vi "Przenies param rej wolna FVG.vi"(7 "Wolna In":T1={"WolnaStart"=FALSE, "WolnaPrzeglad"=FALSE, "Okres"=0.02, "Czas max"=120.0, "WolnaKonfiguracja"=FALSE, "Rej.1"={"Typ rejestracji"=enum."Wprost", "Kanały"=[1], "Opis"="Rej.X", "Aktywny"=FALSE, "Wolna Wykr num"=0}, "Rej.2"={"Typ rejestracji"=enum."Wprost", "Kanały"=[1], "Opis"="Rej.X", "Aktywny"=FALSE, "Wolna Wykr num"=0}, "Rej.3"={"Typ rejestracji"=enum."Wprost", "Kanały"=[1], "Opis"="Rej.X", "Aktywny"=FALSE, "Wolna Wykr num"=0}, "Rej.4"={"Typ rejestracji"=enum."Wprost", "Kanały"=[1], "Opis"="Rej.X", "Aktywny"=FALSE, "Wolna Wykr num"=0}, "Rej.5"={"Typ rejestracji"=enum."Wprost", "Kanały"=[1], "Opis"="Rej.X", "Aktywny"=FALSE, "Wolna Wykr num"=0}, "Rej.6"={"Typ rejestracji"=enum."Wprost", "Kanały"=[1], "Opis"="Rej.X", "Aktywny"=FALSE, "Wolna Wykr num"=0}, "Rej.7"={"Typ rejestracji"=enum."Wprost", "Kanały"=[1], "Opis"="Rej.X", "Aktywny"=FALSE, "Wolna Wykr num"=0}, "Rej.8"={"Typ rejestracji"=enum."Wprost", "Kanały"=[1], "Opis"="Rej.X", "Aktywny"=FALSE, "Wolna Wykr num"=0}} {"Rej.8"."Wolna Wykr num" items=["Brak", "Wykres 1", "Wykres 2", "Wykres 3", "Wykres 4"]; "Rej.7"."Wolna Wykr num" items=["Brak", "Wykres 1", "Wykres 2", "Wykres 3", "Wykres 4"]; "Rej.6"."Wolna Wykr num" items=["Brak", "Wykres 1", "Wykres 2", "Wykres 3", "Wykres 4"]; "Rej.5"."Wolna Wykr num" items=["Brak", "Wykres 1", "Wykres 2", "Wykres 3", "Wykres 4"]; "Rej.4"."Wolna Wykr num" items=["Brak", "Wykres 1", "Wykres 2", "Wykres 3", "Wykres 4"]; "Rej.3"."Wolna Wykr num" items=["Brak", "Wykres 1", "Wykres 2", "Wykres 3", "Wykres 4"]; "Rej.2"."Wolna Wykr num" items=["Brak", "Wykres 1", "Wykres 2", "Wykres 3", "Wykres 4"]; "Rej.1"."Wolna Wykr num" items=["Brak", "Wykres 1", "Wykres 2", "Wykres 3", "Wykres 4"]}, 8 "error in (no error)":errorcluster, 10 "Start In":bool, 11 "Akcja":T5) -> (0 "error out":errorcluster, 2 "Start Out":bool, 3 "Restart Out":bool, 6 "Wolna Out":T1={"WolnaStart"=FALSE, "WolnaPrzeglad"=FALSE, "Okres"=0.02, "Czas max"=120.0, "WolnaKonfiguracja"=FALSE, "Rej.1"={"Typ rejestracji"=enum."Wprost", "Kanały"=[1], "Opis"="Rej.X", "Aktywny"=FALSE, "Wolna Wykr num"=0}, "Rej.2"={"Typ rejestracji"=enum."Wprost", "Kanały"=[1], "Opis"="Rej.X", "Aktywny"=FALSE, "Wolna Wykr num"=0}, "Rej.3"={"Typ rejestracji"=enum."Wprost", "Kanały"=[1], "Opis"="Rej.X", "Aktywny"=FALSE, "Wolna Wykr num"=0}, "Rej.4"={"Typ rejestracji"=enum."Wprost", "Kanały"=[1], "Opis"="Rej.X", "Aktywny"=FALSE, "Wolna Wykr num"=0}, "Rej.5"={"Typ rejestracji"=enum."Wprost", "Kanały"=[1], "Opis"="Rej.X", "Aktywny"=FALSE, "Wolna Wykr num"=0}, "Rej.6"={"Typ rejestracji"=enum."Wprost", "Kanały"=[1], "Opis"="Rej.X", "Aktywny"=FALSE, "Wolna Wykr num"=0}, "Rej.7"={"Typ rejestracji"=enum."Wprost", "Kanały"=[1], "Opis"="Rej.X", "Aktywny"=FALSE, "Wolna Wykr num"=0}, "Rej.8"={"Typ rejestracji"=enum."Wprost", "Kanały"=[1], "Opis"="Rej.X", "Aktywny"=FALSE, "Wolna Wykr num"=0}} {"Rej.8"."Wolna Wykr num" items=["Brak", "Wykres 1", "Wykres 2", "Wykres 3", "Wykres 4"]; "Rej.7"."Wolna Wykr num" items=["Brak", "Wykres 1", "Wykres 2", "Wykres 3", "Wykres 4"]; "Rej.6"."Wolna Wykr num" items=["Brak", "Wykres 1", "Wykres 2", "Wykres 3", "Wykres 4"]; "Rej.5"."Wolna Wykr num" items=["Brak", "Wykres 1", "Wykres 2", "Wykres 3", "Wykres 4"]; "Rej.4"."Wolna Wykr num" items=["Brak", "Wykres 1", "Wykres 2", "Wykres 3", "Wykres 4"]; "Rej.3"."Wolna Wykr num" items=["Brak", "Wykres 1", "Wykres 2", "Wykres 3", "Wykres 4"]; "Rej.2"."Wolna Wykr num" items=["Brak", "Wykres 1", "Wykres 2", "Wykres 3", "Wykres 4"]; "Rej.1"."Wolna Wykr num" items=["Brak", "Wykres 1", "Wykres 2", "Wykres 3", "Wykres 4"]})   [LabVIEW 2013]
doc: "Use this template to build a VI to use as a subVI."
uses:
  Kontrolki/FVGs/FVG akwizycje akcje.ctl
  Kontrolki/GUI/Rejestracja_wolna.ctl
  Kontrolki/GUI/RejWol_konfig.ctl
  Kontrolki/GUI/RejWol_typ.ctl
  Kontrolki/GUI/Wolna_WykrNum.ctl
panel:
  out "Śledzenie Out":enum16{"Obwiednia", "Migawka"}(ring)
  in  "Śledzenie In":enum16{"Obwiednia", "Migawka"}(ring)
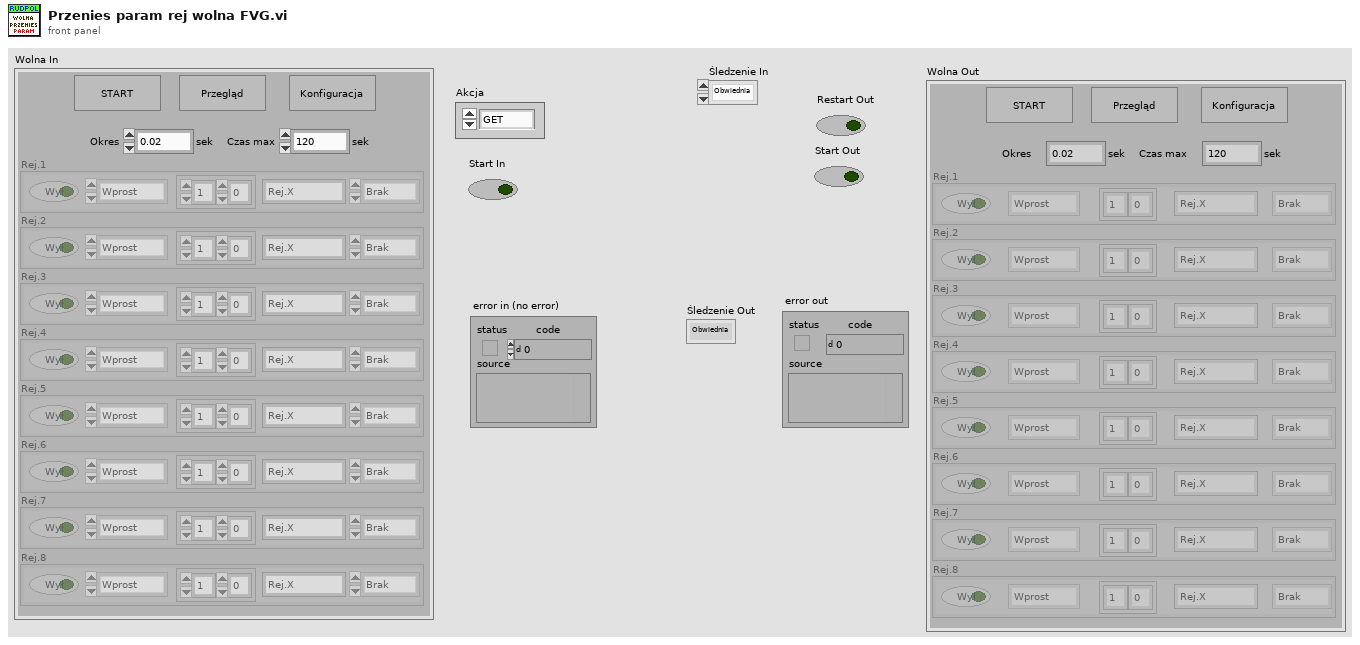
[diagram p1: front panel]
types:
  T1 = typedef "Rejestracja_wolna.ctl" = cluster{"WolnaStart":bool, "WolnaPrzeglad":bool, "Okres":dbl, "Czas max":dbl, "WolnaKonfiguracja":bool, "Rej.1":T2, "Rej.2":T2, "Rej.3":T2, "Rej.4":T2, "Rej.5":T2, "Rej.6":T2, "Rej.7":T2, "Rej.8":T2}
  T2 = typedef "RejWol_konfig.ctl" = cluster{"Typ rejestracji":T3, "Kanały":i32[], "Opis":string, "Aktywny":bool, "Wolna Wykr num":T4}
  T3 = typedef "RejWol_typ.ctl" = enum16{"Wprost", "Moduł", "Kwadrat", "Iloczyn", "Faza"}
  T4 = typedef "Wolna_WykrNum.ctl" = u16
  T5 = typedef "FVG akwizycje akcje.ctl" = enum16{"GET", "GETr", "SET"}
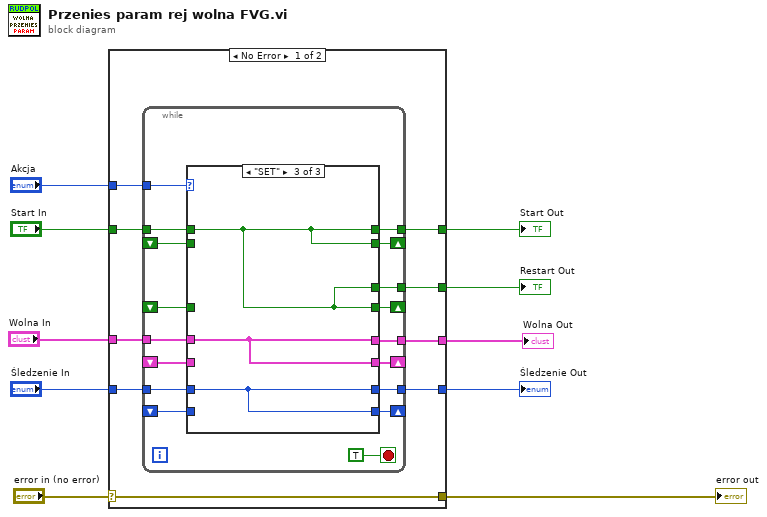
[diagram p0: block diagram]
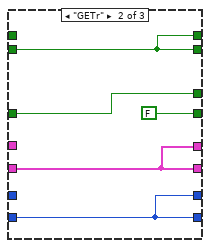
[diagram p3: hidden frame]
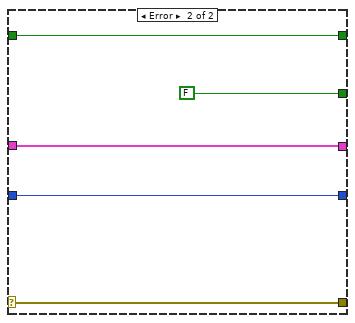
[diagram p4: hidden frame]
diagram:
  n1 = case shown="No Error" "error in (no error)" {
    selector: "error in (no error)" -> [w19 w53]
    tunnel: [w19 w53] -> w9
    tunnel: "Akcja" -> [w18 _]
    tunnel: "Start In" -> [w17 w52]
    tunnel: "Wolna In" -> [w16 w50]
    tunnel: "Śledzenie In" -> [w15 w49]
    tunnel: [w14 w52] -> w5
    tunnel: [w13 FALSE ("Start In")] -> w4
    tunnel: [w12 w50] -> w1
    tunnel: [w11 w49] -> w3
    frame No Error {
      n2 = while {
        tunnel: w18 -> [w35]
        tunnel: w17 -> [w34]
        tunnel: w16 -> [w33]
        tunnel: w15 -> [w32]
        shift-right: [w31] -> _
        shift-left: _ -> [w30]
        shift-right: [w29] -> _
        shift-left: _ -> [w25]
        shift-right: [w28] -> _
        shift-left: _ -> [w24]
        shift-right: [w27] -> _
        shift-left: _ -> [w22]
        tunnel: [w26] -> w14
        tunnel: [w23] -> w12
        tunnel: [w21] -> w11
        tunnel: [w20] -> w13
        stop <- TRUE stop-if-true
        n3 = case shown="\"SET\"" w35 {
          tunnel: w34 -> [_ _ w46]
          tunnel: w33 -> [_ _ w47]
          tunnel: w32 -> [_ _ w48]
          tunnel: [w40 w43 w46] -> w31
          tunnel: w30 -> [w40 w43 _]
          tunnel: [w37 FALSE ("Start In") w46] -> w29
          tunnel: [w39 w45 w47] -> w28
          tunnel: [w38 w44 w48] -> w27
          tunnel: [w40 w43 w46] -> w26
          tunnel: w25 -> [w37 w41 _]
          tunnel: w24 -> [w39 w45 _]
          tunnel: [w39 w45 w47] -> w23
          tunnel: w22 -> [w38 w44 _]
          tunnel: [w38 w44 w48] -> w21
          tunnel: [w37 w41 w46] -> w20
          frame "GET", Default {
          }
          frame "GETr" {
          }
          frame "SET" {
          }
        }
      }
    }
    frame Error {
    }
  }
  "error out" <- w9
  "Restart Out" <- w4
  "Śledzenie Out" <- w3
  "Start Out" <- w5
  "Wolna Out" <- w1
